vi "GetSetLiveAux.vi"(0 "VISA resource name":refnum<visa-resource-name>, 5 "get/set":T2=enum."set", 7 "Live Aux Number (1-8)":T1=1 min=1 max=8, 9 "State (o=off, 1=on)":i8 min=0 max=1 step=1, 11 "error in":errorcluster) -> (4 "VISA resource name out":refnum<visa-resource-name>, 6 "Live Aux State (0=off, 1=on)":i32, 8 "Enabled? (0=disabled, 1=enabled)":i32, 15 "error out":errorcluster)   [LabVIEW 2023, in "Thermotron 8800.lvlib"]
doc: "LAUX\nCommand name: Send or load live auxiliary settings\nCommand type: Variable\nDescription: Unlike standard auxiliary relays, live auxiliaries can be enabled without the 8800 being in run mode. The query command asks the 8800 for the status of the selected live\nauxiliary. The operation command allows you to set the live auxiliary variables.\nQuery syntax: LAUXaux?\nOperation syntax: LAUXaux, state\nWhere:\naux live auxiliary number (1 through 8)\nstate 0 (off) or 1 (on)\nQuery example 1: LAUX2?\n8800 response: 0, 0 (Live auxiliary 2 is not on, and it is not enabled.)\nQuery example 2: LAUX1?\n8800 response: 0, 1 (Live auxiliary 1 is not on, but it is enabled.)\nOperation example: LAUX2, 1\n8800 response: 0 (The 8800 changed live auxiliary 2 to be on, but only if it is enabled.)"
uses:
  Thermotron 8800.lvlib
  Private/get set.ctl
  Private/Live Aux Number.ctl
panel:
  out "read buffer":string
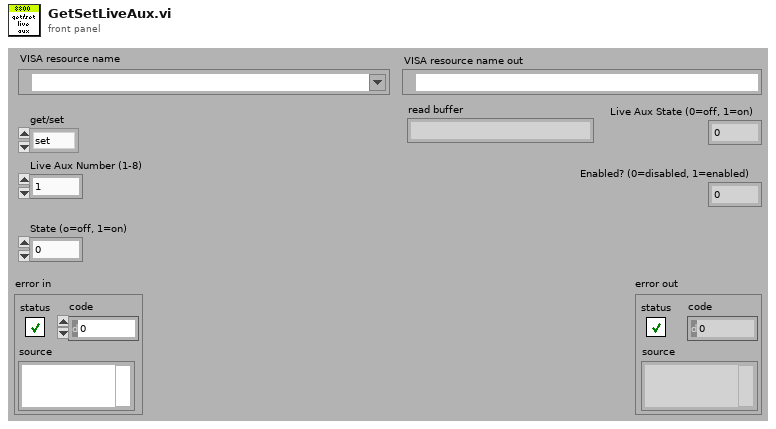
[diagram p1: front panel]
types:
  T1 = typedef "Thermotron 8800.lvlib/Live Aux Number.ctl" = i8
  T2 = typedef "Thermotron 8800.lvlib/get set.ctl" = enum16{"get", "set"}
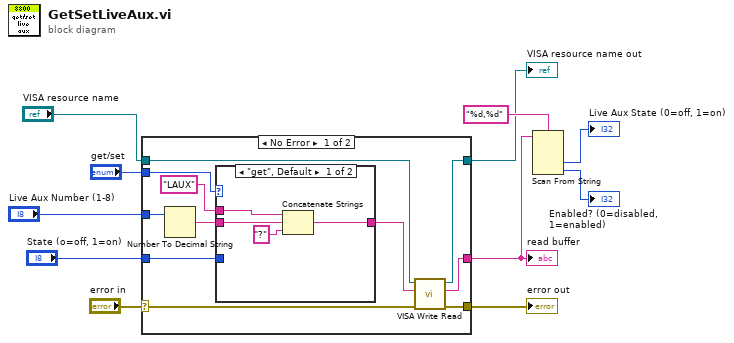
[diagram p0: block diagram]
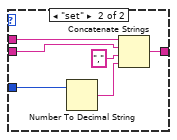
[diagram p2: hidden frame]
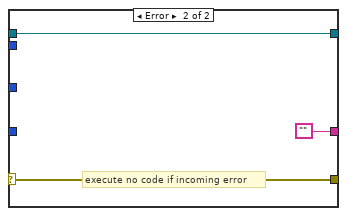
[diagram p3: hidden frame]
diagram:
  n1 = case shown="No Error" "error in" {
    selector: "error in" -> [w20 w35]
    tunnel: [w18 w35] -> w6
    tunnel: [w19 w34] -> w5
    tunnel: "VISA resource name" -> [w21 w34]
    tunnel: "get/set" -> [w16 _]
    tunnel: [w17 ""] -> w2
    tunnel: "Live Aux Number (1-8)" -> [w13 _]
    tunnel: "State (o=off, 1=on)" -> [w14 _]
    frame No Error {
      n2 = Number To Decimal String(number=w13) -> (decimal integer string=w12:string)  [unwired: 1 in]
      n3 = case shown="\"get\", Default" w16 {
        tunnel: "LAUX" ("8800 Command") -> [w25 w32]
        tunnel: [w26 w31] -> w22
        tunnel: w14 -> [_ w30]
        tunnel: w12 -> [w23 w27]
        frame "get", Default {
          n4 = Concatenate Strings(w25, w23, "?" ("8800 Command")) -> (w26:string)
        }
        frame "set" {
          n5 = Number To Decimal String(number=w30) -> (decimal integer string=w28:string)  [unwired: 1 in]
          n6 = Concatenate Strings(w32, w27, "," ("string"), w28) -> (w31:string)
        }
      }
      n7 = call "VISA Write Read.vi"("error in (no error)"=w20, "8800 Command"=w22, "VISA Refnum in"=w21) -> ("error out"=w18:errorcluster, "read buffer"=w17:string, "VISA Refnum out"=w19:refnum<visa-resource-name>)  [unwired: 6 in]
    }
    frame Error {
      # "execute no code if incoming error"
    }
  }
  "VISA resource name out" <- w5
  "error out" <- w6
  "read buffer" <- w2
  n8 = Scan From String(format string="%d,%d", input string=w2) -> (output 1=→"Live Aux State (0=off, 1=on)":i32, output 2=→"Enabled? (0=disabled, 1=enabled)":i32)  [unwired: 4 in, 3 out]
